vi "getStatusEotBkwd.vi"(8 "error in":errorcluster, 9 "Get Stus EOT BKWD in":bool=TRUE, 10 "axis in":u8, 11 "connection ID":refnum<k5>) -> (0 "error out":errorcluster, 1 "Get Stus EOT BKWD out":bool=TRUE, 2 "axis out":u8, 3 "connection ID":refnum<k5>)   [LabVIEW 2016]
panel:
  in  "Get Command":string="com.attocube.amc.status.getStatusEotBkwd"
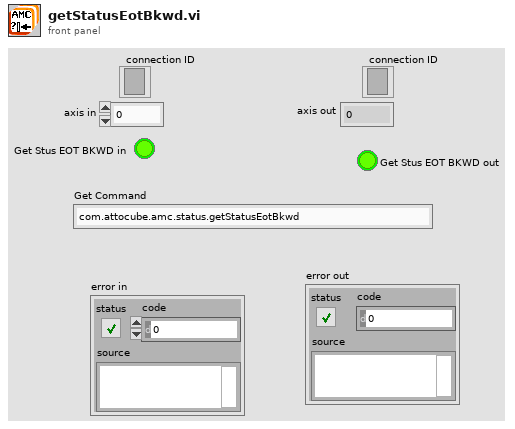
[diagram p1: front panel]
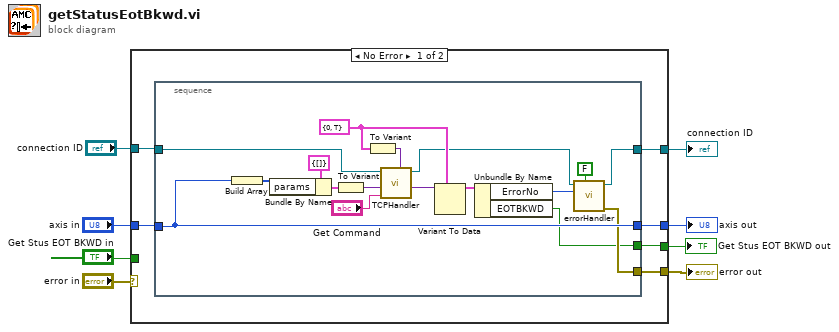
[diagram p0: block diagram]
diagram:
  n1 = case shown="No Error" "error in" {
    selector: "error in" -> [_ w33]
    tunnel: "axis in" -> [w9 w35]
    tunnel: [w14 w33] -> w7
    tunnel: [w12 w35] -> w6
    tunnel: [w11 w34] -> w5
    tunnel: [w13 w32] -> w4
    tunnel: "connection ID" -> [w10 w32]
    tunnel: "Get Stus EOT BKWD in" -> [_ w34]
    frame No Error {
      n2 = stacked-sequence {
        tunnel: [w15] -> w13
        tunnel: w10 -> [w21]
        tunnel: w9 -> [w23]
        tunnel: [w23] -> w12
        tunnel: [w18] -> w11
        tunnel: [w22] -> w14
        frame #0 {
          w19 = cluster{"ErrorNo":i32, "EOTBKWD":bool} {"ErrorNo"=0, "EOTBKWD"=TRUE} ("input cluster")
          n3 = Build Array(w23) -> (w27:u8[])
          n4 = Bundle By Name(cluster=cluster{"params":i32[]} {"params"=[]} ("input cluster"), "params"=w27) -> (w28:cluster{"params":i32[]})
          n5 = To Variant(anything=w28) -> (Variant=w29:variant)
          n6 = To Variant(anything=w19) -> (Variant=w20:variant)
          n7 = call "TCPHandler.vi"("result Types"=w20, "method"="Get Command", "params"=w29, "connection ID"=w21) -> ("result"=w25:variant, "connection ID"=w16:refnum<k5>)  [unwired: 5 in, 1 out]
          n8 = Variant To Data(type=w19, Variant=w25) -> (data=w30:cluster{"ErrorNo":i32, "EOTBKWD":bool})  [unwired: 1 in, 1 out]
          n9 = Unbundle By Name(w30) -> ("ErrorNo"=w31:i32, "EOTBKWD"=w18:bool)
          n10 = call "errorHandler.vi"("show popup"=FALSE, "error number"=w31, "connection ID"=w16) -> ("error out"=w22:errorcluster, "connection ID"=w15:refnum<k5>)  [unwired: 7 in]
        }
      }
    }
    frame Error {
    }
  }
  "error out" <- w7
  "axis out" <- w6
  "Get Stus EOT BKWD out" <- w5
  "connection ID" <- w4
